vi "BSA Initial vi.vi"() -> ()   [LabVIEW 2014]
doc: "I. Description:\nThis example demonstrates how to acquire a continuous amount of data (Waveform) using the DAQ device's internal clock.\n\nII. Instructions for Running:\n1. Create an analog input voltage channel.\n2. Set the rate for the sample clock. Additionally, define the sample mode to be continuous.\n3. Call the Start VI to start the acquisition.\n4. Read the waveform data in a loop until the user hits the stop button or an error occurs.\nNote: This example reads data from one or more channels and returns an array of data. Use the Index Array function to access an individual channel of data.\n5. Call the Clear Task VI to clear the Task.\n6. Use the popup dialog box to display an error if any.\n\nIV. I/O Connections Overview:\nMake sure your signal input terminal matches the Physical Channel I/O Control. For further connection information, refer to your hardware reference manual."
uses:
  <vilib>/DAQmx/create/channels.llb/DAQmx Create Channel (AI-Voltage-Basic).vi
  <vilib>/DAQmx/configure/timing.llb/DAQmx Timing (Sample Clock).vi
  <vilib>/Waveform/WDTOps.llb/WDT Waveform to XY Pairs DBL.vi
  <vilib>/DAQmx/read.llb/DAQmx Read (Analog 1D Wfm NChan NSamp).vi
  <vilib>/addons/Digital Filter Design/Design.llb/DFD IIR Notch Peak Design by BW.vi
  <vilib>/addons/Digital Filter Design/Process.llb/DFD Filtering (Wfm NChan).vi
  <vilib>/measure/mamon.llb/Waveform Peak Detection for 1 Chan.vi
  <vilib>/addons/Digital Filter Design/NI_DigFilterLicensed.lvlib
  <vilib>/measure/NI_MAPro.lvlib
  <vilib>/Analysis/NI_AAL_SigProc.lvlib
panel:
  in  "peaks/valleys":enum32{"Peaks", "Valleys"}(ring)
  in  "width":i32=3 min=3
  in  "threshold 2":dbl format="%0.2f"
  out "XY Graph":cluster{"Locations":dbl[], "Amplitudes":dbl[]}[](graph)
  in  "PD width":i32=3 min=3
  in  "threshold":dbl format="%0.2f"
  out "#Peaks Found\n in 2 sec":i32
  out "ECG":waveform(dbl)(graph)
  out "Heart Rate \n(beats/min)":dbl
  out "Sound":waveform(dbl)(graph)
  out "2 peaks found?":bool
  in  "Samples to Read":i32=1000
  in  "Physical Channel":tag="Dev1/ai0"
  in  "Minimum Value":dbl=-10.0 caption="Min (V)" format="%0.2f"
  in  "Maximum Value":dbl=10.0 caption="Max (V)" format="%0.2f"
  in  "stop":bool
  in  "Sample Rate":dbl=10000.0 caption="Sample Rate (Hz)" format="%0.2f"
  # "For instructions, select Help>>Show Context Help"
  # "Thresholding Parameters"
  # "Channel Parameters"
  # "Make sure your figures are all on the same scale!!"
  # "A/D\nconversion"
  # "Timing Parameters"
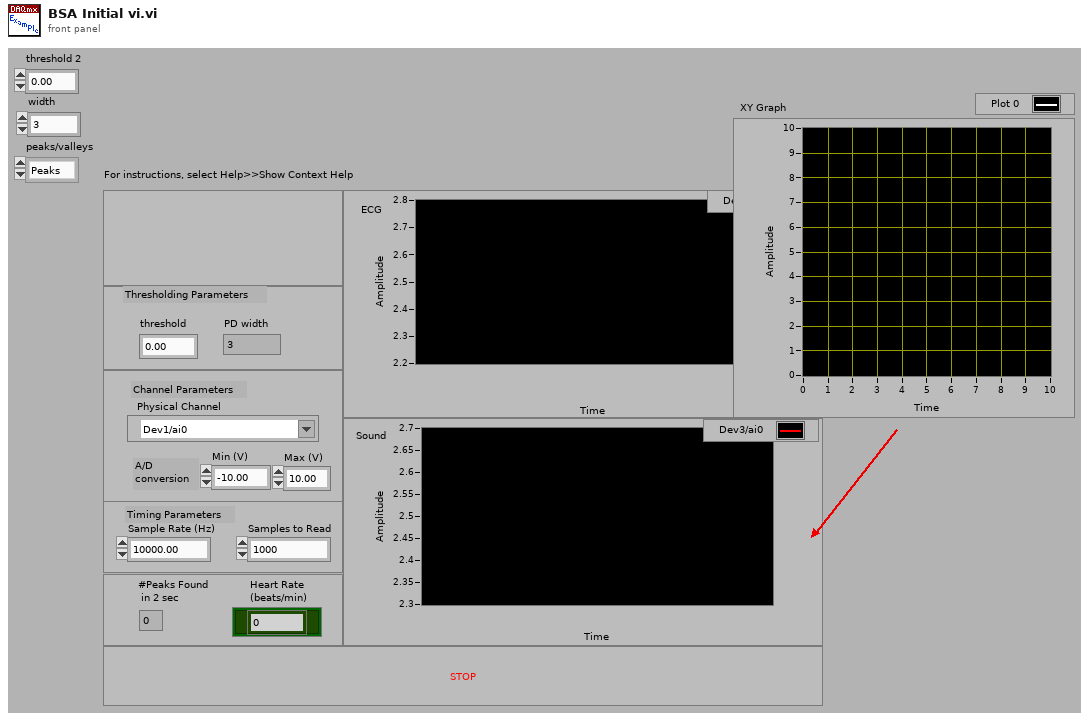
[diagram p1: front panel]
types:
  T1 = typedef "NI_DigFilterLicensed.lvlib/DFD Filter Obj.ctl" = cluster{"mSRate_Fs":dbl, "mSRate_Version":string, "mSRate_Comments":string, "mSRate_OrgCoef":T2, "mSRate_CurCoef":T2, "mSRate_Quantized?":bool, "mSRate_QCoef":T2, "mSRate_QSettings":T4[], "mSRate_Order":i32, "mSRate_Scaling":cluster{"mSRate_ScaleByPowerOf2?":bool, "mSRate_ScaleType":T6}}
  T2 = typedef "NI_DigFilterLicensed.lvlib/DFD Filter Coef.ctl" = cluster{"type":T3, "gain":dbl, "coef a (k)":dbl[], "coef b (v)":dbl[]}
  T3 = typedef "NI_DigFilterLicensed.lvlib/DFD Filter Structure Type Selector.ctl" = enum16{"Undefined", "FIR Direct Form", "FIR Direct Form Transposed", "FIR Symmetric", "FIR Antisymmetric", "IIR Direct Form I", "IIR Direct Form I Transposed", "IIR Direct Form II", "IIR Direct Form II Transposed", "IIR Cascaded Second Order Sections Form I", "IIR Cascaded Second Order Sections Form I Transposed", "IIR Cascaded Second Order Sections Form II", "IIR Cascaded Second Order Sections Form II Transposed", "Lattice Allpass (basic sections)", "Lattice Allpass (one multiplier sections)", "Lattice Allpass (normalized sections)", "Lattice AR (basic sections)", "Lattice AR (one multiplier sections)", "Lattice AR (normalized sections)", "Lattice MA (minimum phase)", "Lattice MA (maximum phase)", "Lattice ARMA (basic sections)", "Lattice ARMA (one multiplier sections)", "Lattice ARMA (normalized sections)"}
  T4 = typedef "NI_DigFilterLicensed.lvlib/dfd_Internal Quantization Settings.ctl" = cluster{"source":T5, "wl":i16, "iwl":i16, "overflow mode":enum16{"Saturation", "Wrap"}, "rounding mode":enum16{"Nearest", "Truncation"}, "signed?":bool}
  T5 = typedef "NI_DigFilterLicensed.lvlib/dfd_Internal Quantization Srcs.ctl" = u16
  T6 = typedef "NI_DigFilterLicensed.lvlib/DFD Coef Norm Type.ctl" = enum16{"No Norm", "Time Domain 1-Norm", "Time Domain 2-Norm", "Time Domain Inf-Norm"}
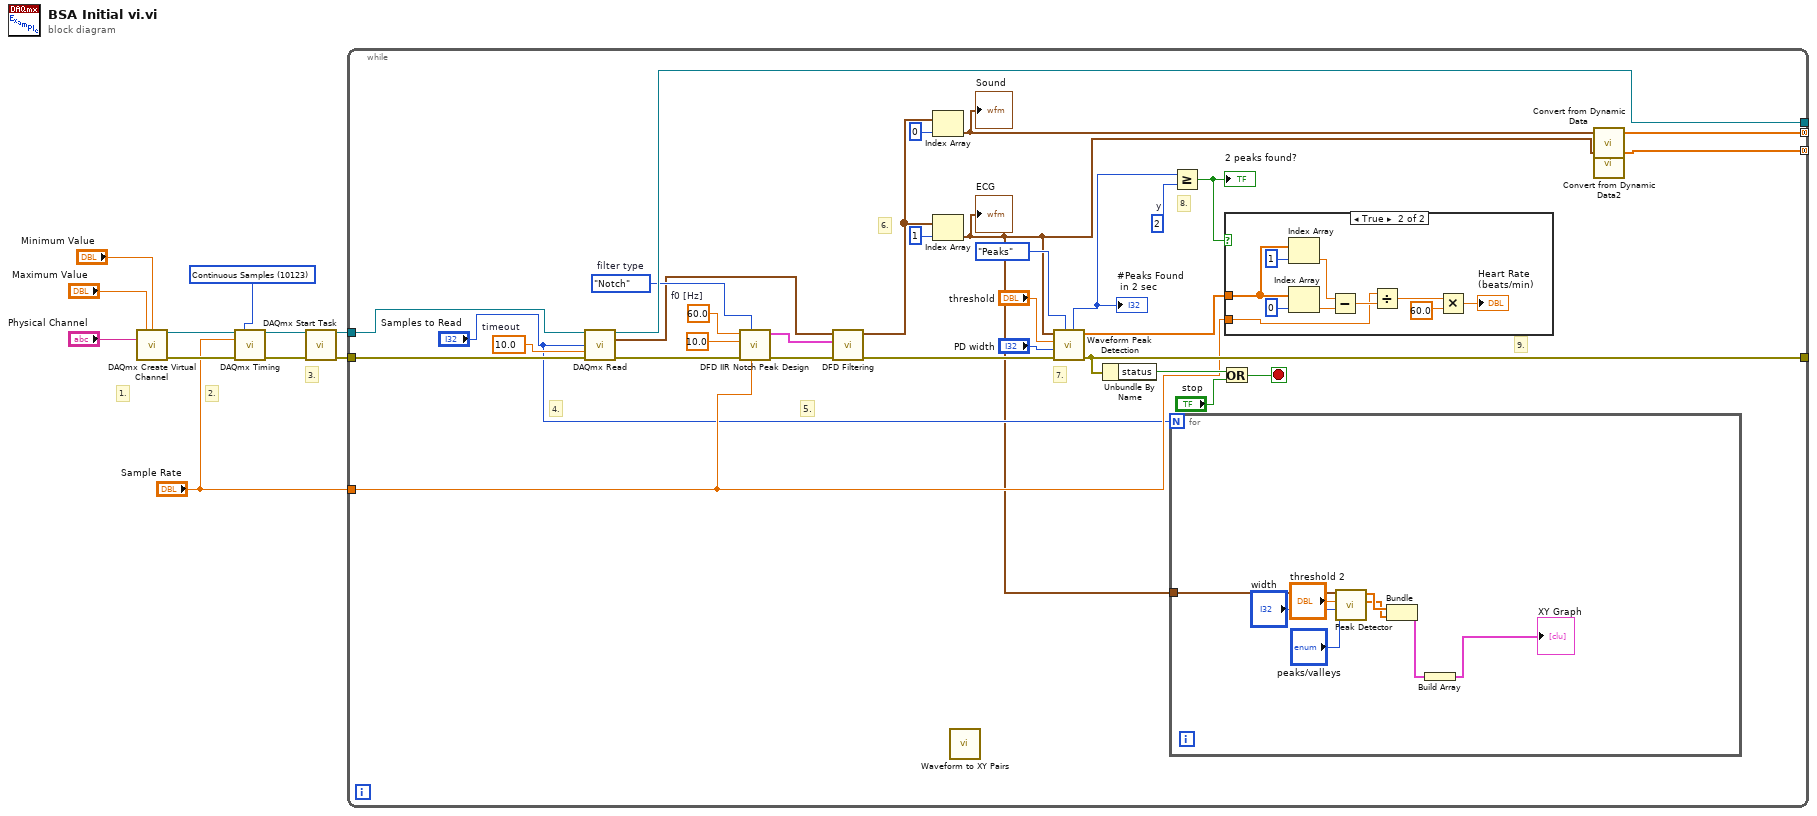
[diagram p0: block diagram]
diagram:
  w4 = 10123 items=["Finite Samples"=10178, "Continuous Samples"=10123] ("sample mode")
  # "2."
  # "1."
  # "3."
  n1 = call-poly <vilib>:"DAQmx Create Virtual Channel.vi"("maximum value"="Maximum Value", "minimum value"="Minimum Value", "physical channels"="Physical Channel") -> ("task out"=w7:refnum<k21>, "error out"=w9:errorcluster)  [unwired: 6 in, 5 out]
  n2 = call-poly <vilib>:"DAQmx Timing.vi"("task/channels in"=w7, "sample mode"=w4, "rate"="Sample Rate", "error in"=w9) -> ("task out"=w3:refnum<k21>, "error out"=w2:errorcluster)  [unwired: 3 in, 7 out]
  n3 = call <vilib>:"DAQmx Start Task.vi"("task/channels in"=w3, "error in"=w2) -> ("task out"=w6:refnum<k21>, "error out"=w8:errorcluster)  [unwired: 12 out]
  n4 = while {
    tunnel: w8 -> [w43]
    tunnel: w6 -> [w42]
    tunnel: [w41] -> _
    tunnel: [w20] -> _
    tunnel: "Sample Rate" -> [w16]
    tunnel: [w15] -> _ mode=concatenating
    tunnel: [w14] -> _ mode=concatenating
    stop <- w39 stop-if-true
    w18 = 2  # y
    w34 = enum16{"Notch", "Peak"}."Notch"  # filter type
    w35 = 60.0  # f0 [Hz]
    w37 = 10.0  # timeout
    # "9."
    # "8."
    # "7."
    # "6."
    # "5."
    # "4."
    n5 = call-poly <vilib>:"DAQmx Read.vi"("task/channels in"=w42, "number of samples per channel"="Samples to Read", "timeout"=w37, "error in"=w43) -> ("task out"=w41:refnum<k21>, "data"=w25:waveform(dbl)[], "error out"=w32:errorcluster)  [unwired: 9 out]
    n6 = call-poly <vilib>:"DFD IIR Notch Peak Design.vi"("fs [Hz]"=w16, "filter type"=w34, "error in (no error)"=w32, "Df [Hz]"=10.0 ("Q factor"), "f0 [Hz]"=w35) -> ("error out"=w31:errorcluster, "filter out"=w33:T1)  [unwired: 1 in, 4 out]
    n7 = call-poly <vilib>:"DFD Filtering.vi"("error in (no error)"=w31, "filter"=w33, "signal in"=w25) -> ("error out"=w21:errorcluster, "signal out"=w22:waveform(dbl)[])  [unwired: 1 in, 6 out]
    n8 = Index Array(array=w22, index=0) -> (element=w24:waveform(dbl))
    "Sound" <- w24
    n9 = Index Array(array=w22, index=1) -> (element=w12:waveform(dbl))
    "ECG" <- w12
    n10 = call-poly <vilib>:"Waveform to XY Pairs.vi"() -> ()  [unwired: 9 in, 3 out]
    n11 = call-poly <vilib>:"Waveform Peak Detection.vi"("peaks/valleys"=enum32{"Peaks", "Valleys"}."Peaks", "error in"=w21, "width"="PD width", "threshold"="threshold", "Signal In"=w12) -> ("error out"=w20:errorcluster, "Locations"=w30:dbl[], "# found"=w19:i32)  [unwired: 2 in, 2 out]
    "#Peaks Found\n in 2 sec" <- w19
    n12 = Unbundle By Name(w20) -> ("status"=w40:bool)
    n13 = for {
      N: "Samples to Read" -> [_]
      tunnel: w12 -> [w51]
      n14 = call <vilib>:"Peak Detector.vi"("peaks/valleys"="peaks/valleys", "width"="width", "threshold"="threshold 2", "X"=w51) -> ("Amplitudes"=w46:dbl[], "Locations"=w47:dbl[])  [unwired: 3 in, 3 out]
      n15 = Bundle("Locations"=w47, "Amplitudes"=w46) -> (w45:cluster{"Locations":dbl[], "Amplitudes":dbl[]})  [unwired: 1 in]
      n16 = Build Array(w45) -> (→"XY Graph":cluster{"Locations":dbl[], "Amplitudes":dbl[]}[])
    }
    n17 = Greater Or Equal?(x=w19, y=w18) -> (x >= y?=w17:bool)
    "2 peaks found?" <- w17
    n18 = Or(x=w40, y="stop") -> (x .or. y?=w39:bool)
    n19 = case shown="True" w17 {
      tunnel: w30 -> [_ w56]
      tunnel: w16 -> [_ w52]
      frame False {
      }
      frame True {
        n20 = Index Array(array=w56, index=1) -> (element=w58:dbl)
        n21 = Index Array(array=w56, index=0) -> (element=w57:dbl)
        n22 = Subtract(x=w58, y=w57) -> (x-y=w53:dbl)
        n23 = Divide(x=w52, y=w53) -> (x/y=w59:dbl)
        n24 = Multiply(x=w59, y=60.0) -> (x*y=→"Heart Rate \n(beats/min)":dbl)
      }
    }
    n25 = call "Convert from Dynamic Data"("Dynamic Data Type"=w24) -> ("Array"=w15:dbl[])  [unwired: 3 out]
    n26 = call "Convert from Dynamic Data2"("Dynamic Data Type"=w12) -> ("Array"=w14:dbl[])  [unwired: 3 out]
  }
